vi "Read one digital line v1.0.2.vi"() -> ()   [LabVIEW 2014]
uses:
  <vilib>/DAQmx/create/channels.llb/DAQmx Create Channel (DI-Digital Input).vi
  <vilib>/DAQmx/read.llb/DAQmx Read (Digital Bool 1Line 1Point).vi
panel:
  in  "lines":tag="Dev1/port0/line1"
  in  "quit":bool
  out "Line":bool
  out "error out":errorcluster
  in  "rate":dbl=1000.0 format="%0.2f"
  in  "active edge":i32(ring)=10280 items=["Rising"=10280, "Falling"=10171]
  in  "samples per channel":i32=1000
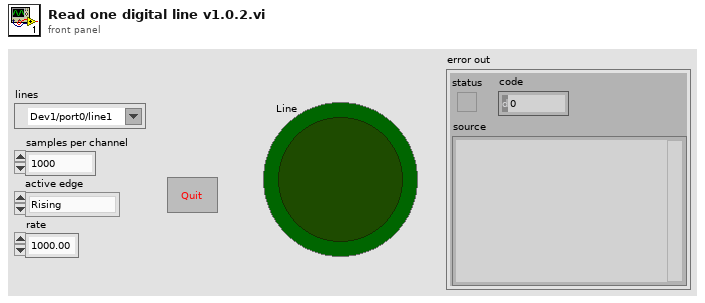
[diagram p1: front panel]
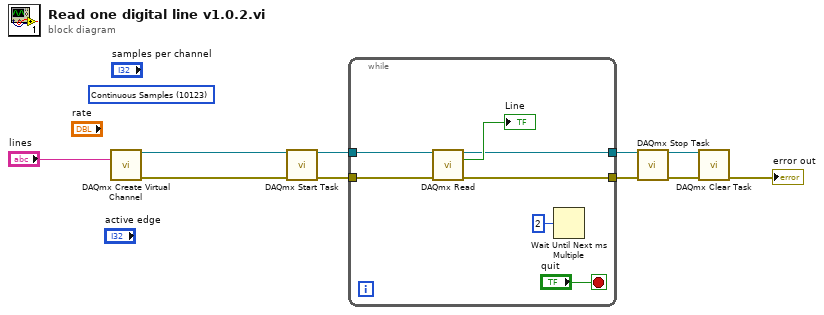
[diagram p0: block diagram]
diagram:
  (unwired) 10123 items=["Finite Samples"=10178, "Continuous Samples"=10123, "Hardware Timed Single Point"=12522] ("sample mode")
  n1 = call-poly <vilib>:"DAQmx Create Virtual Channel.vi"("lines"="lines") -> ("task out"=w3:refnum<k21>, "error out"=w2:errorcluster)  [unwired: 13 in]
  n2 = call <vilib>:"DAQmx Start Task.vi"("task/channels in"=w3, "error in"=w2) -> ("task out"=w7:refnum<k21>, "error out"=w5:errorcluster)  [unwired: 12 in]
  n3 = while {
    tunnel: w7 -> [w16]
    tunnel: [w15] -> w6
    tunnel: w5 -> [w14]
    tunnel: [w13] -> w4
    stop <- "quit" stop-if-true
    n4 = call-poly <vilib>:"DAQmx Read.vi"("task/channels in"=w16, "error in"=w14) -> ("task out"=w15:refnum<k21>, "data"=→"Line":bool, "error out"=w13:errorcluster)  [unwired: 11 in]
    n5 = Wait Until Next ms Multiple(millisecond multiple=u32 2) -> ()  [unwired: 1 out]
  }
  n6 = call <vilib>:"DAQmx Stop Task.vi"("task/channels in"=w6, "error in"=w4) -> ("task out"=w10:refnum<k21>, "error out"=w9:errorcluster)  [unwired: 12 in]
  n7 = call <vilib>:"DAQmx Clear Task.vi"("task in"=w10, "error in"=w9) -> ("error out"=→"error out":errorcluster)  [unwired: 13 in]
